vi "Configure Frequency Slew Rate.vi"(0 "VISA resource name":refnum<visa-resource-name>, 5 "Frequency Slew Rate Mode (0: Fixed)":i32(ring) items=["Fixed", "Step", "Pulse", "List"], 7 "Frequency Slew Rate (1e-3 Hz)":dbl=0.001, 9 "Triggered Frequency Slew Rate (1e-3 Hz)":dbl=0.001, 11 "error in (no error)":errorcluster) -> (4 "VISA resource name out":refnum<visa-resource-name>, 15 "error out":errorcluster)   [LabVIEW 2013, in "Cal Inst.lvlib" / "California Instruments iX Series.lvlib"]
doc: "Configures the frequency slew rate, mode and triggered slew rate."
uses:
  California Instruments iX Series.lvlib
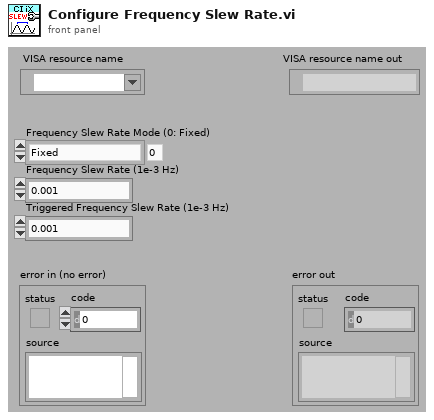
[diagram p1: front panel]
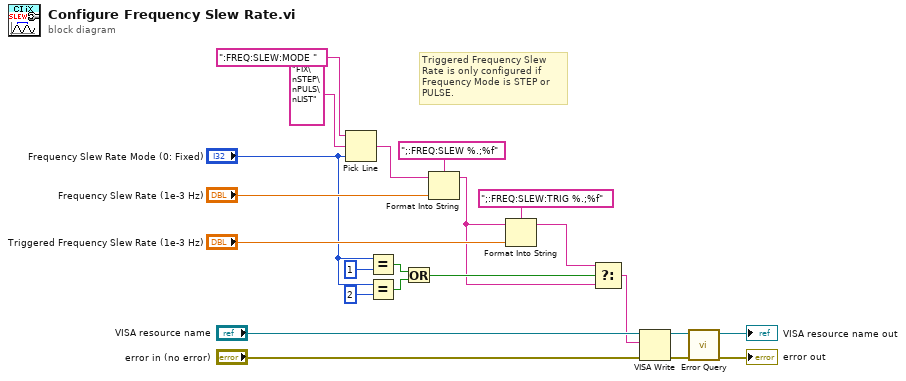
[diagram p0: block diagram]
diagram:
  # "Triggered Frequency Slew Rate is only configured if Frequency Mode is STEP or PULSE."
  n1 = Pick Line(string ("")=":FREQ:SLEW:MODE ", multi-line string="FIX\nSTEP\nPULS\nLIST", line index="Frequency Slew Rate Mode (0: Fixed)") -> (output string=w14:string)
  n2 = Equal?(x="Frequency Slew Rate Mode (0: Fixed)", y=1) -> (x = y?=w6:bool)
  n3 = Equal?(x="Frequency Slew Rate Mode (0: Fixed)", y=2) -> (x = y?=w5:bool)
  n4 = Or(x=w6, y=w5) -> (x .or. y?=w4:bool)
  n5 = Format Into String(format string=";:FREQ:SLEW %.;%f", initial string=w14, "Frequency Slew Rate (1e-3 Hz)") -> (resulting string=w3:string)  [unwired: 1 in, 1 out]
  n6 = Format Into String(format string=";:FREQ:SLEW:TRIG %.;%f", initial string=w3, "Triggered Frequency Slew Rate (1e-3 Hz)") -> (resulting string=w2:string)  [unwired: 1 in, 1 out]
  n7 = Select(t=w2, s=w4, f=w3) -> (s? t:f=w1:string)
  n8 = VISA Write(VISA resource name="VISA resource name", write buffer=w1, error in (no error)="error in (no error)") -> (VISA resource name out=w18:refnum<visa-resource-name>, error out=w21:errorcluster)  [unwired: 1 out]
  n9 = call "Error Query.vi"("error in (no error)"=w21, "VISA resource name"=w18) -> ("error out"=→"error out":errorcluster, "VISA resource name out"=→"VISA resource name out":refnum<visa-resource-name>)  [unwired: 6 in, 2 out]
